vi "3-2.vi"() -> ()   [LabVIEW 2019, in "3.lvlib"]
uses:
  3.lvlib
  <vilib>/Utility/file.llb/Read Delimited Spreadsheet (string).vi
panel:
  out "life support rating":u32
  out "oxygen generator rating":u32
  out "CO2 scrubber rating":u32
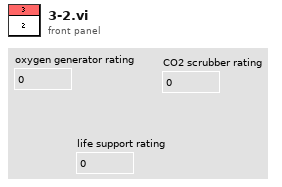
[diagram p1: front panel]
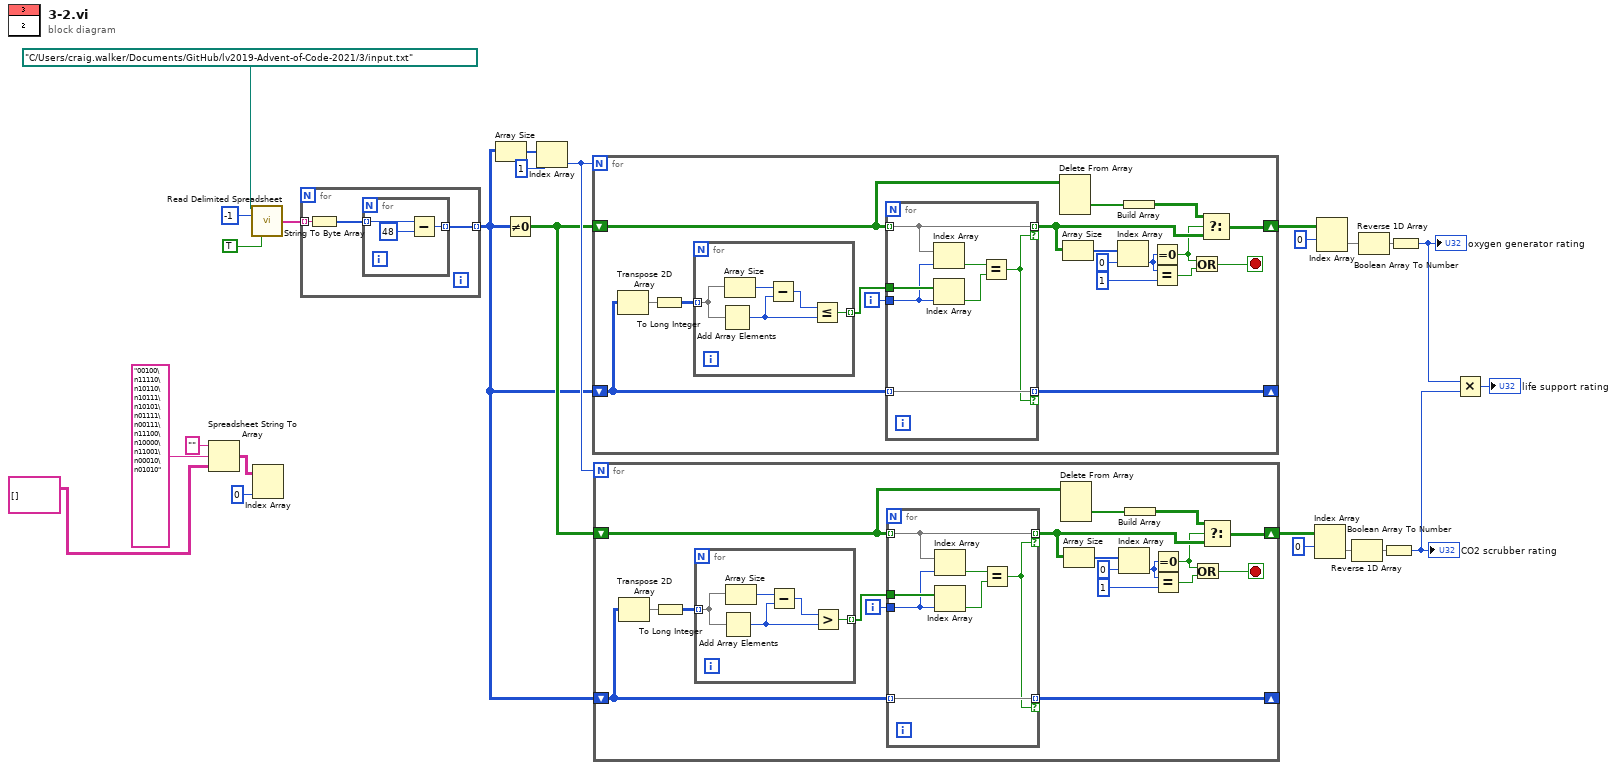
[diagram p0: block diagram]
diagram:
  n1 = Spreadsheet String To Array(format string="", spreadsheet string="00100\n11110\n10110\n10111\n10101\n01111\n00111\n11100\n10000\n11001\n00010\n01010", array type (2D Dbl)=string[][] [] ("format string")) -> (array=w17:string[][])  [unwired: 1 in]
  n2 = call-poly <vilib>:"Read Delimited Spreadsheet.vi"("file path (dialog if empty)"=path "C:/Users/craig.walker/Documents/GitHub/lv2019-Advent-of-Code-2021/3/input.txt", "number of rows (all:-1)"=-1, "transpose? (F)"=TRUE) -> ("first row"=w1:string[])  [unwired: 7 in, 5 out]
  n3 = Index Array(array=w17, index (col)=0 ("disabled index (col)")) -> ()  [unwired: 1 in, 1 out]
  n4 = for {
    tunnel: w1 -> [w28] mode=indexing
    tunnel: [w26] -> w11 mode=indexing
    n5 = String To Byte Array(string=w28) -> (unsigned byte array=w27:u8[])
    n6 = for {
      tunnel: w27 -> [w31] mode=indexing
      tunnel: [w29] -> w26 mode=indexing
      n7 = Subtract(x=w31, y=u8 48) -> (x-y=w29:u8)
    }
  }
  n8 = Array Size(array=w11) -> (size(s)=w15:i32[])
  n9 = Not Equal To 0?(x=w11) -> (x != 0?=w12:bool[][])
  n10 = Index Array(array=w15, index=1) -> (element=w13:i32)
  n11 = for {
    N: w13 -> [_]
    shift-right: [w42] -> w22
    shift-left: w12 -> [w36]
    shift-right: [w32] -> _
    shift-left: w11 -> [w33]
    i -> [w43]
    stop <- w44 stop-if-true
    n12 = Transpose 2D Array(2D array=w33) -> (transposed array=w34:u8[][])
    n13 = To Long Integer(number=w34) -> (32bit integer=w37:i32[][])
    n14 = for {
      tunnel: w37 -> [w54] mode=indexing
      tunnel: [w50] -> w35 mode=indexing
      n15 = Add Array Elements(numeric array=w54) -> (sum=w51:i32)
      n16 = Array Size(array=w54) -> (size(s)=w53:i32)
      n17 = Subtract(x=w53, y=w51) -> (x-y=w52:i32)
      n18 = Less Or Equal?(x=w52, y=w51) -> (x <= y?=w50:bool)
    }
    n19 = for {
      tunnel: w36 -> [w58] mode=indexing
      tunnel: w35 -> [w61]
      tunnel: [w58] -> w41 mode=indexing if=w55
      tunnel: w43 -> [w57]
      tunnel: w33 -> [w56] mode=indexing
      tunnel: [w56] -> w32 mode=indexing if=w55
      n20 = Index Array(array=w58, index=w57) -> (element=w59:bool)
      n21 = Index Array(array=w61, index=w57) -> (element=w60:bool)
      n22 = Equal?(x=w59, y=w60) -> (x = y?=w55:bool)
    }
    n23 = Delete From Array(array=w36) -> (deleted portion=w39:bool[])  [unwired: 3 in, 1 out]
    n24 = Array Size(array=w41) -> (size(s)=w49:i32[])
    n25 = Index Array(array=w49, index=0) -> (element=w46:i32)
    n26 = Build Array(w39) -> (w38:bool[][])
    n27 = Equal To 0?(x=w46) -> (x = 0?=w40:bool)
    n28 = Equal?(x=w46, y=1) -> (x = y?=w45:bool)
    n29 = Or(x=w40, y=w45) -> (x .or. y?=w44:bool)
    n30 = Select(t=w38, s=w40, f=w41) -> (s? t:f=w42:bool[][])
  }
  n31 = for {
    N: w13 -> [_]
    shift-right: [w72] -> w9
    shift-left: w12 -> [w66]
    shift-right: [w63] -> _
    shift-left: w11 -> [w64]
    i -> [w73]
    stop <- w74 stop-if-true
    n32 = Transpose 2D Array(2D array=w64) -> (transposed array=w65:u8[][])
    n33 = To Long Integer(number=w65) -> (32bit integer=w67:i32[][])
    n34 = for {
      tunnel: w67 -> [w84] mode=indexing
      tunnel: [w80] -> w62 mode=indexing
      n35 = Add Array Elements(numeric array=w84) -> (sum=w81:i32)
      n36 = Array Size(array=w84) -> (size(s)=w83:i32)
      n37 = Subtract(x=w83, y=w81) -> (x-y=w82:i32)
      n38 = Greater?(x=w82, y=w81) -> (0:w80:bool)
    }
    n39 = for {
      tunnel: w66 -> [w88] mode=indexing
      tunnel: w62 -> [w91]
      tunnel: [w88] -> w71 mode=indexing if=w85
      tunnel: w73 -> [w87]
      tunnel: w64 -> [w86] mode=indexing
      tunnel: [w86] -> w63 mode=indexing if=w85
      n40 = Index Array(array=w88, index=w87) -> (element=w89:bool)
      n41 = Index Array(array=w91, index=w87) -> (element=w90:bool)
      n42 = Equal?(x=w89, y=w90) -> (x = y?=w85:bool)
    }
    n43 = Delete From Array(array=w66) -> (deleted portion=w69:bool[])  [unwired: 3 in, 1 out]
    n44 = Array Size(array=w71) -> (size(s)=w79:i32[])
    n45 = Index Array(array=w79, index=0) -> (element=w76:i32)
    n46 = Build Array(w69) -> (w68:bool[][])
    n47 = Equal To 0?(x=w76) -> (x = 0?=w70:bool)
    n48 = Equal?(x=w76, y=1) -> (x = y?=w75:bool)
    n49 = Or(x=w70, y=w75) -> (x .or. y?=w74:bool)
    n50 = Select(t=w68, s=w70, f=w71) -> (s? t:f=w72:bool[][])
  }
  n51 = Index Array(array=w9, index (row)=0) -> (element=w8:bool[])  [unwired: 1 in]
  n52 = Index Array(array=w22, index (row)=0) -> (element=w5:bool[])  [unwired: 1 in]
  n53 = Reverse 1D Array(array=w8) -> (reversed array=w7:bool[])
  n54 = Reverse 1D Array(array=w5) -> (reversed array=w6:bool[])
  n55 = Boolean Array To Number(Boolean array=w7) -> (number=w3:u32)
  "CO2 scrubber rating" <- w3
  n56 = Boolean Array To Number(Boolean array=w6) -> (number=w4:u32)
  "oxygen generator rating" <- w4
  n57 = Multiply(x=w4, y=w3) -> (x*y=→"life support rating":u32)
